vi "GetParam.vi"(8 "error in (no error)":errorcluster, 11 "Reconstruct_from_patches_2d in":refnum<class "Reconstruct_from_patches_2d.lvclass">) -> (0 "error out":errorcluster, 2 "image_size":cluster{"image_height":i32, "image_width":i32}, 3 "Reconstruct_from_patches_2d out":refnum<class "Reconstruct_from_patches_2d.lvclass">)   [LabVIEW 2020, in "Reconstruct_from_patches_2d.lvclass"]
uses:
  Reconstruct_from_patches_2d.lvclass
  Reconstruct_from_patches_2d.lvclass/Reconstruct_from_patches_2d.ctl
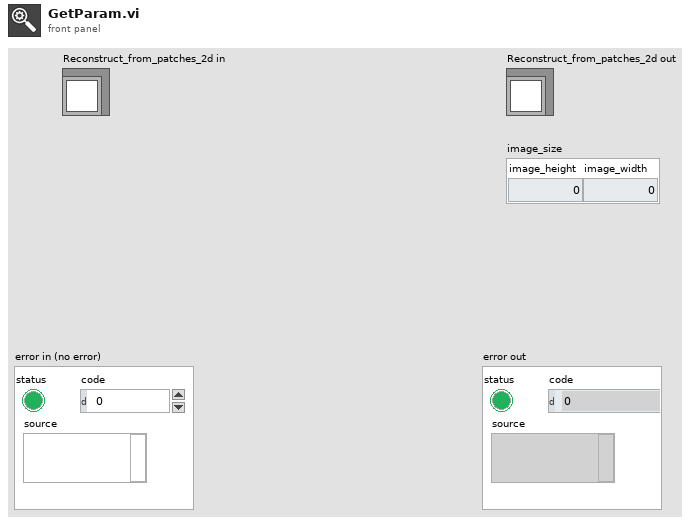
[diagram p1: front panel]
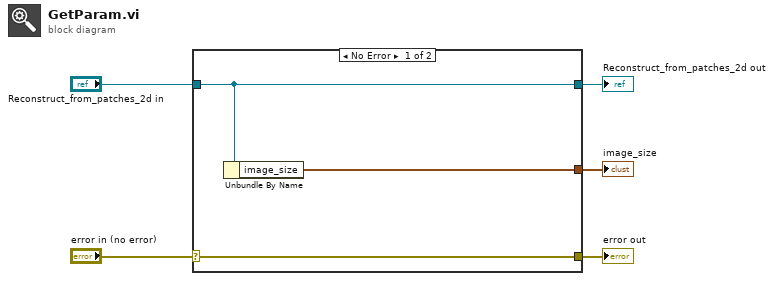
[diagram p0: block diagram]
diagram:
  n1 = case shown="No Error" "error in (no error)" {
    selector: "error in (no error)" -> [w8 w9]
    tunnel: [w8 w9] -> w4
    tunnel: [w7 w10] -> w2
    tunnel: "Reconstruct_from_patches_2d in" -> [w7 w10]
    tunnel: [w6 _] -> w1
    frame No Error {
      n2 = Unbundle By Name(w7) -> ("image_size"=w6:cluster{"image_height":i32, "image_width":i32})
    }
    frame Error {
    }
  }
  "error out" <- w4
  "Reconstruct_from_patches_2d out" <- w2
  "image_size" <- w1
